vi "lvstyx_get_usb_connection.vi"(2 "error in (no error)":errorcluster) -> (0 "error out":errorcluster, 1 "connection ptr":u32 format="%08x")   [LabVIEW 2010, in "lib1299.lvlib"]
uses:
  lib1299.lvlib
  cstyx/win32/cstyx.dll
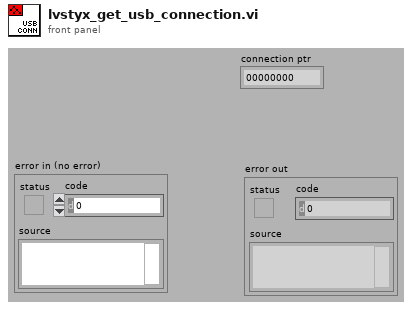
[diagram p1: front panel]
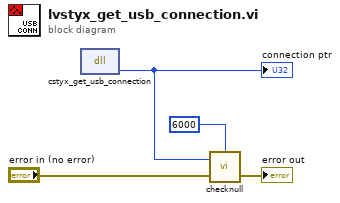
[diagram p0: block diagram]
diagram:
  n1 = dll-call lib="C:/work/ads1299evm/lib_1299/Styx/cstyx/win32/cstyx.dll" fn="cstyx_get_usb_connection"() -> (w4:u32)  [unwired: 3 in, 2 out]
  "connection ptr" <- w4
  n2 = call "checknull.vi"("error in (no error)"="error in (no error)", "ptr"=w4, "error code"=6000) -> ("error out"=→"error out":errorcluster)  [unwired: 2 in]
